vi "Update Conjunctions.vi"(9 "Destination Map in":map{string, string[]}(c390), 10 "Module Map in":map{string, refnum<class "Module.lvclass">}(c390), 11 "Conjunctions in":string[](array[string])) -> (2 "Destination Map out":map{string, string[]}(c390), 3 "Module Map out":map{string, refnum<class "Module.lvclass">}(c390))   [LabVIEW 2021]
uses:
  Day 20/Module/Module.lvclass
  Day 20/Conjunction/Conjunction.lvclass
  C:/Projects/LabVIEWAdventOfCode2023/Day 20/Module/Module.lvclass
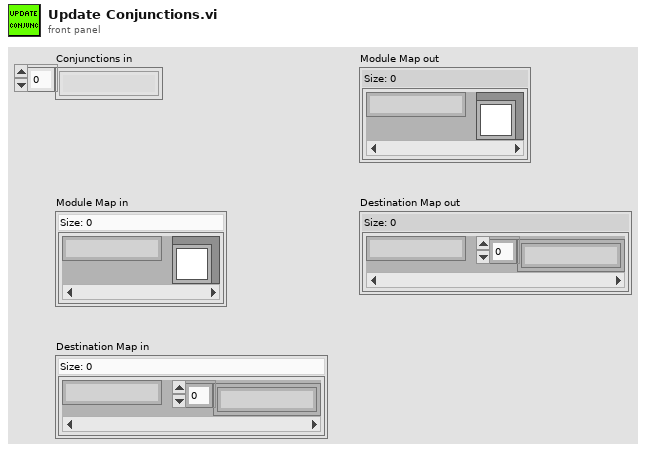
[diagram p1: front panel]
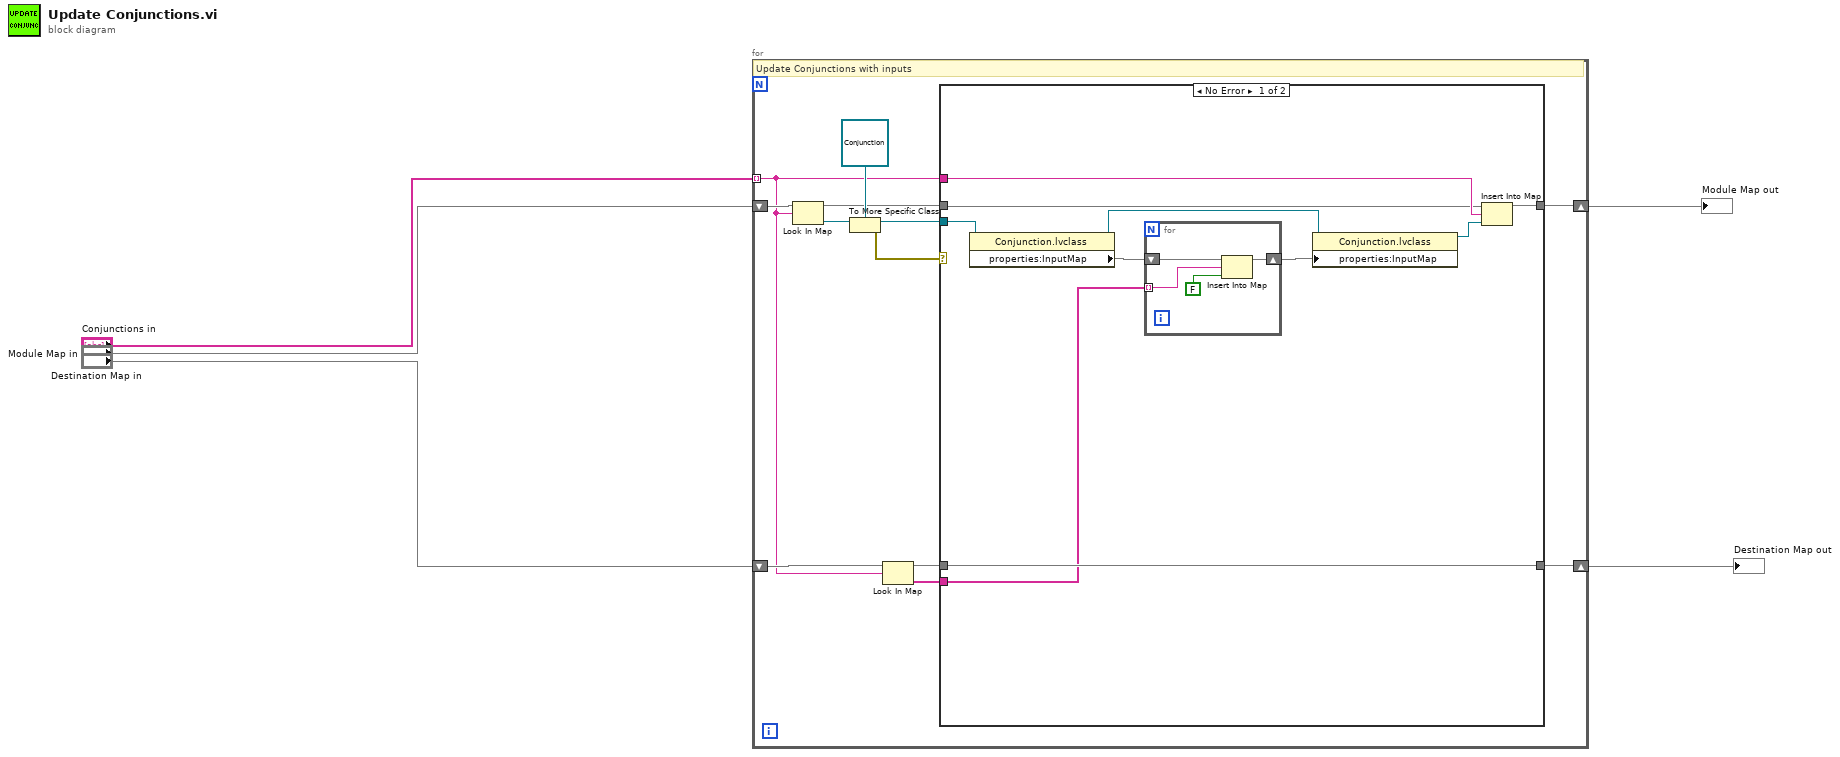
[diagram p0: block diagram]
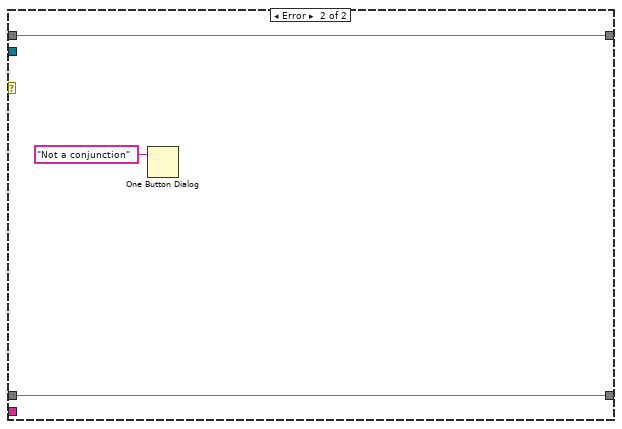
[diagram p2: hidden frame]
diagram:
  n1 = for {
    tunnel: "Conjunctions in" -> [w6] mode=indexing
    shift-right: [w10] -> w4
    shift-left: "Module Map in" -> [w11]
    shift-right: [w8] -> w5
    shift-left: "Destination Map in" -> [w9]
    # "Update Conjunctions with inputs"
    n2 = Look In Map(map=w11, key=w6) -> (value=w14:refnum<class "Module.lvclass">)  [unwired: 1 in, 1 out]
    n3 = To More Specific Class(target class=refnum<class "Conjunction.lvclass"> refnum ("Conjunction.lvclass"), reference=w14) -> (specific class reference=w13:refnum<class "Conjunction.lvclass">, error out=w12:errorcluster)  [unwired: 1 in]
    n4 = Look In Map(map=w9, key=w6) -> (value=w7:string[])  [unwired: 1 in, 1 out]
    n5 = case shown="No Error" w12 {
      tunnel: w13 -> [w24 _]
      tunnel: w11 -> [w17 w31]
      tunnel: [w19 w31] -> w10
      tunnel: w9 -> [w25 w30]
      tunnel: [w25 w30] -> w8
      tunnel: w7 -> [w23 _]
      tunnel: w6 -> [w18 _]
      frame No Error {
        n6 = property class="Conjunction.lvclass"(reference=w24) -> (reference out=w20:refnum<class "Conjunction.lvclass">, "properties:InputMap"=w22:map{string, bool})  [unwired: 1 in, 1 out]
        n7 = for {
          tunnel: w23 -> [w28] mode=indexing
          shift-right: [w26] -> w21
          shift-left: w22 -> [w29]
          n8 = Insert Into Map(map in=w29, key=w28, value=FALSE) -> (map out=w26:map{string, bool})  [unwired: 2 out]
        }
        n9 = property class="Conjunction.lvclass"(reference=w20, "properties:InputMap"=w21) -> (reference out=w16:refnum<class "Conjunction.lvclass">)  [unwired: 1 in, 1 out]
        n10 = Insert Into Map(map in=w17, key=w18, value=w16) -> (map out=w19:map{string, refnum<class "Module.lvclass">})  [unwired: 2 out]
      }
      frame Error {
        n11 = One Button Dialog(message="Not a conjunction") -> ()  [unwired: 1 in, 1 out]
      }
    }
  }
  "Destination Map out" <- w5
  "Module Map out" <- w4
